vi "Copy .LLB to NI VeriStand dir.vi"(5 "Files Generated by Build":path[](array[path]), 6 "Top Level/Always Included VIs":path[](array[path]), 7 "Destination Path":path, 8 "error in (no error)":errorcluster, 9 "Target Name":string, 10 "Build Specification Name":string, 11 "Project Path":path) -> (0 "error out":errorcluster)   [LabVIEW 2024]
doc: "This VI is called after each run of a build specification. The VI will copy the generated LLB (Engine or System Explorer) into the VeriStand Custom Device folder (...\\Documents\\National Instruments\\NI VeriStand 2013...)."
uses:
  NationalInstruments.VeriStand
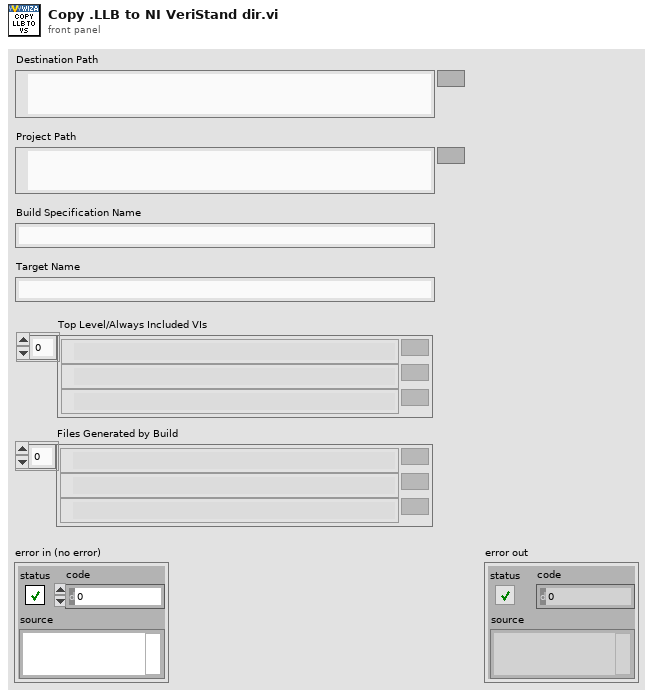
[diagram p1: front panel]
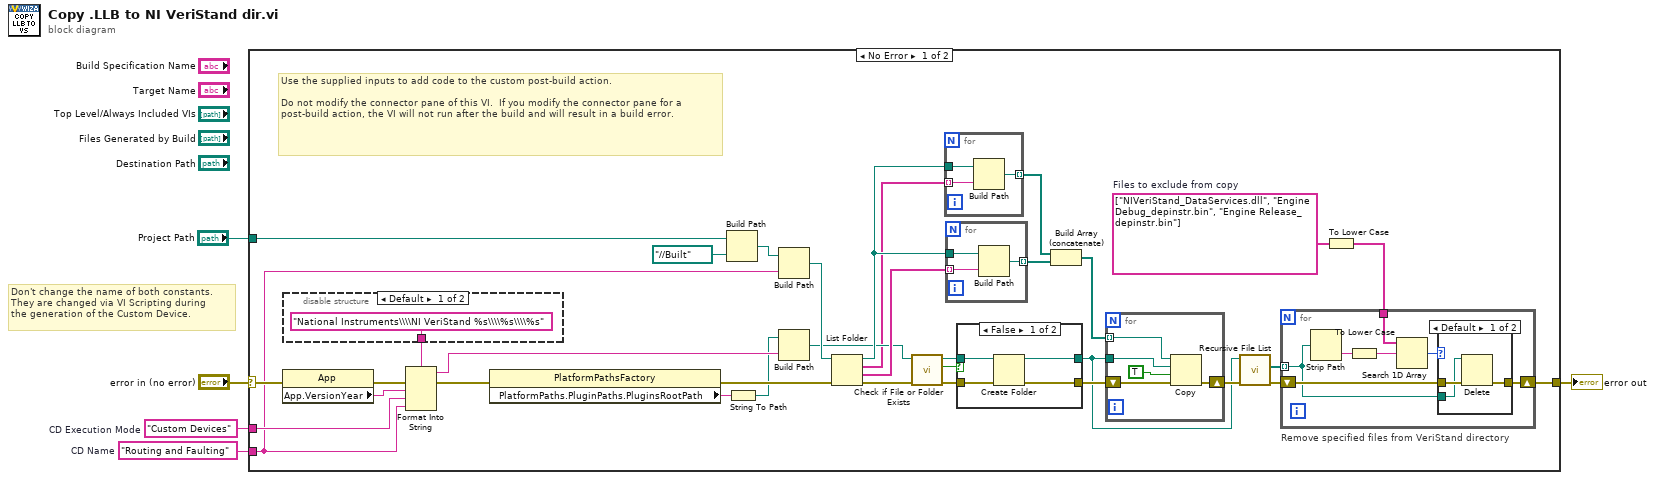
[diagram p0: block diagram]
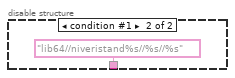
[diagram p2: hidden frame]
diagram:
  w2 = "Routing and Faulting"  # CD Name
  w3 = "Custom Devices"  # CD Execution Mode
  # "Don't change the name of both constants.\nThey are changed via VI Scripting during\nthe generation of the Custom Device."
  n1 = case shown="No Error" "error in (no error)" {
    selector: "error in (no error)" -> [w22 w70]
    tunnel: [w10 w70] -> w1
    tunnel: "Project Path" -> [w19 _]
    tunnel: w3 -> [w23 _]
    tunnel: w2 -> [w21 _]
    frame No Error {
      w16 = string[] ["NIVeriStand_DataServices.dll", "Engine Debug_depinstr.bin", "Engine Release_depinstr.bin"]  # Files to exclude from copy
      # "Use the supplied inputs to add code to the custom post-build action.\n\nDo not modify the connector pane of this VI.  If you modify the connector pane for a post-build action, the VI will not run after the build and will result in a build error."
      n2 = property class="App"(error in=w22) -> (error out=w27:errorcluster, "App.VersionYear"=w26:string)  [unwired: 1 in, 1 out]
      n3 = disable-structure shown="Default" {
        disable-tunnel: ["National Instruments\\\\NI VeriStand %s\\\\%s\\\\%s" ("name or relative path") "lib64//niveristand%s//%s//%s" ("name or relative path")] -> w25
        frame condition #0 (active) {
        }
        frame condition #1 {
        }
      }
      n4 = Format Into String(format string=w25, error in=w27, w26, w23, w21) -> (resulting string=w28:string, error out=w9:errorcluster)  [unwired: 1 in]
      n5 = property class="PlatformPathsFactory"(error in=w9) -> (error out=w8:errorcluster, "PlatformPaths.PluginPaths.PluginsRootPath"=w7:string)  [unwired: 1 in, 1 out]
      n6 = Build Path(base path=w19, name or relative path=path "../../Built") -> (appended path=w29:path)
      n7 = String To Path(string=w7) -> (path=w6:path)
      n8 = Build Path(base path=w29, name or relative path=w21) -> (appended path=w31:path)
      n9 = Build Path(base path=w6, name or relative path=w28) -> (appended path=w24:path)
      n10 = List Folder(path=w31, error in=w8) -> (path out=w33:path, filenames=w17:string[], folder names=w34:string[], error out=w30:errorcluster)  [unwired: 2 in]
      n11 = call <vilib>:"Check if File or Folder Exists.vi"("error in (no error)"=w30, "path"=w24) -> ("error out"=w35:errorcluster, "file or folder exists?"=w37:bool, "dup path"=w36:path)  [unwired: 7 in]
      n12 = for {
        tunnel: w17 -> [w68] mode=indexing
        tunnel: w33 -> [w69]
        tunnel: [w67] -> w39 mode=indexing
        n13 = Build Path(base path=w69, name or relative path=w68) -> (appended path=w67:path)
      }
      n14 = for {
        tunnel: w34 -> [w65] mode=indexing
        tunnel: w33 -> [w66]
        tunnel: [w64] -> w32 mode=indexing
        n15 = Build Path(base path=w66, name or relative path=w65) -> (appended path=w64:path)
      }
      n16 = case shown="False" w37 {
        tunnel: w36 -> [w56 w58]
        tunnel: w35 -> [w55 w57]
        tunnel: [w54 w58] -> w11
        tunnel: [w53 w57] -> w18
        frame False {
          n17 = Create Folder(path (use dialog)=w56, error in=w55) -> (created path=w54:path, error out=w53:errorcluster)  [unwired: 1 in, 1 out]
        }
        frame True {
        }
      }
      n18 = Build Array (concatenate)(w39, w32) -> (w38:path[])
      n19 = for {
        tunnel: w38 -> [w60] mode=indexing
        shift-right: [w61] -> w12
        shift-left: w18 -> [w62]
        tunnel: w11 -> [w59]
        n20 = Copy(8:w62, 9:TRUE ("overwrite (F)"), 10:w59, 11:w60) -> (0:w61:errorcluster)  [unwired: 1 in, 2 out]
      }
      n21 = call <vilib>:"Recursive File List.vi"("error in (no error)"=w12, "Folder Path"=w11) -> ("error out"=w15:errorcluster, "All Files in Dir"=w14:path[])  [unwired: 5 in, 3 out]
      n22 = To Lower Case(string=w16) -> (all lower case string=w13:string[])
      n23 = for "Remove specified files from VeriStand directory" {
        shift-right: [w43] -> w10
        shift-left: w15 -> [w45]
        tunnel: w14 -> [w42] mode=indexing
        tunnel: w13 -> [w46]
        n24 = Strip Path(path=w42) -> (name=w48:string)  [unwired: 1 out]
        n25 = To Lower Case(string=w48) -> (all lower case string=w47:string)
        n26 = Search 1D Array(1D array=w46, element=w47) -> (index of element=w44:i32)  [unwired: 1 in]
        n27 = case shown="Default" w44 {
          tunnel: w45 -> [w51 w52]
          tunnel: [w50 w52] -> w43
          tunnel: w42 -> [w49 _]
          frame Default {
            n28 = Delete(path (use dialog)=w49, error in=w51) -> (error out=w50:errorcluster)  [unwired: 3 in, 2 out]
          }
          frame -1 {
          }
        }
      }
    }
    frame Error {
    }
  }
  "error out" <- w1
